vi "Configuration Write Do.vi"(7 "Digit Resolution(5½)":T1=enum."5½", 8 "error in (no error)":errorcluster, 9 "Range":dbl, 10 "Function":T2, 11 "DMM Driver in":refnum<class "DMM Driver.lvclass">) -> (0 "error out":errorcluster, 1 "Success?":bool, 3 "DMM Driver out":refnum<class "DMM Driver.lvclass">)   [LabVIEW 2020, in "DMM.lvlib" / "DMM Driver.lvclass"]
doc: "Configure the DMM Function, Range and Resolution."
uses:
  DMM Driver.lvclass
  Controls/Ctl_Function.ctl
  Controls/Ctl_DigitResolution.ctl
  DMM.lvlib
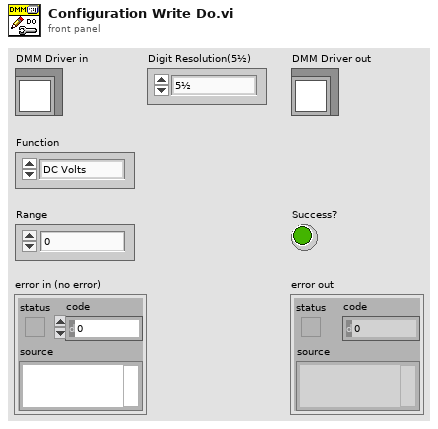
[diagram p1: front panel]
types:
  T1 = typedef "DMM.lvlib/Ctl_DigitResolution.ctl" = enum8{"3½", "4½", "5½", "6½", "7½"}
  T2 = typedef "DMM.lvlib/Ctl_Function.ctl" = enum8{"DC Volts", "AC Volts", "DC Current", "AC Current", "2-wire Resistance", "4-wire Resistance", "Diode", "Frequency", "Period", "AC Volts DC Coupled", "Capacitance", "Inductance", "Temperature"}
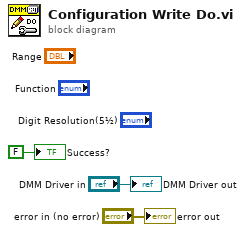
[diagram p0: block diagram]
diagram:
  "error out" <- "error in (no error)"
  "DMM Driver out" <- "DMM Driver in"
  "Success?" <- FALSE ("Success?")
